vi "CAN2.vi"() -> (0 "error out":errorcluster, 1 "CAN 2":T1, 2 "CAN1":T1, 3 "FPGA VI Reference Out":refnum<k20>)   [LabVIEW 2021]
uses:
  <vilib>/FPGAPlugInAG/cRIO-9068/niLvFpga_Open_cRIO-9068.vi
  <vilib>/FPGAPlugInAG/cRIO-9068/niLvFpga_Run_cRIO-9068.vi
  <vilib>/xnet/xnet.llb/XNET Create Session (Frame Input Stream).vi
  <vilib>/xnet/xnet.llb/XNET Create Session (Frame Output Stream).vi
  <vilib>/rvi/interface/nirviOpenFPGA/nirviOpenFPGA.xnode
  FPGA Bitfiles/pv-emulators_FPGATarget_emptyFPGA_z5uule7UYNw.lvbitx
  <vilib>/rvi/interface/nirviMethod/nirviMethod.xnode
  <resource>/objmgr/xnet.rc
panel:
  out "Devices":refnum<k21>[](array[refnum])
  out "iteration":i32
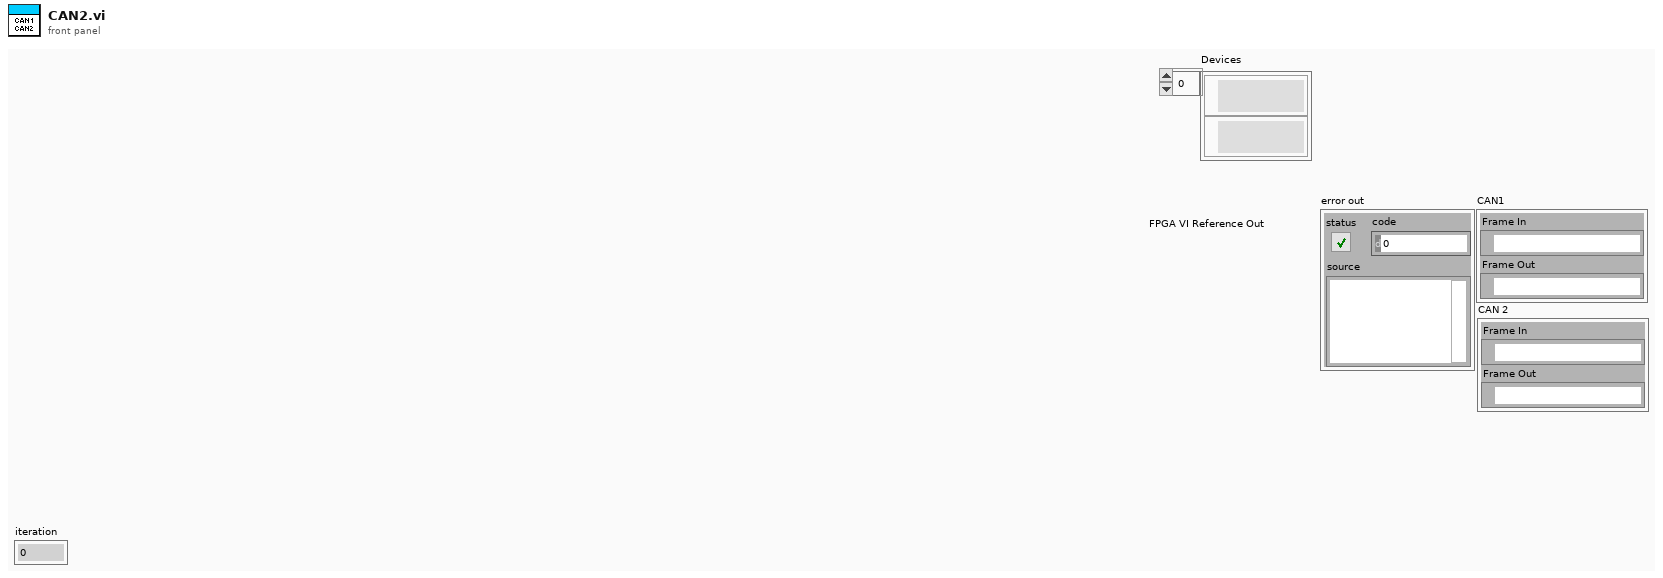
[diagram p1: front panel]
types:
  T1 = cluster{"Frame In":refnum<k21>, "Frame Out":refnum<k21>}
  T2 = cluster{"session out":refnum<k21>, "session out":refnum<k21>}
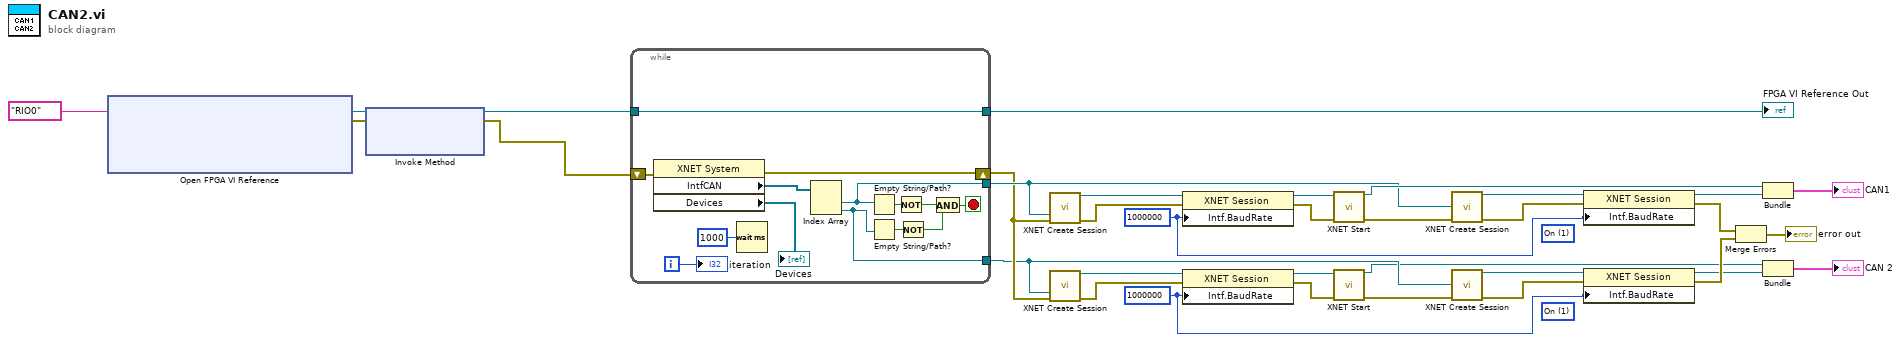
[diagram p0: block diagram]
diagram:
  (unwired) u32 1 items=["Off", "On"] ("Interface:CAN:Termination")
  w4 = u32 1000000 ("y")
  (unwired) u32 1 items=["Off", "On"] ("Interface:CAN:Termination")
  w27 = u32 1000000 ("y")
  n1 = xnode "Open FPGA VI Reference"("resource name"=tag "RIO0") -> ("FPGA VI Reference Out"=w20:refnum<k20>, "error out"=w22:errorcluster)  [unwired: 1 in]
  n2 = xnode "Invoke Method"("FPGA VI Reference In"=w20, "error in"=w22) -> ("FPGA VI Reference Out"=w19:refnum<k20>, "error out"=w18:errorcluster)  [unwired: 1 in]
  n3 = while {
    tunnel: [w41] -> w17
    tunnel: [w45] -> w23
    tunnel: w19 -> [w45]
    shift-right: [w43] -> w16
    shift-left: w18 -> [w44]
    tunnel: [w40] -> w15
    i -> [w47]
    stop <- w35 stop-if-true
    n4 = property class="XNET System"(error in=w44) -> (error out=w43:errorcluster, "IntfCAN"=w42:refnum<k21>[], "Devices"=→"Devices":refnum<k21>[])  [unwired: 1 in, 1 out]
    n5 = Wait (ms)(milliseconds to wait=u32 1000) -> ()  [unwired: 1 out]
    n6 = Index Array(array=w42) -> (element #1=w41:refnum<k21>, element #2=w40:refnum<k21>)  [unwired: 2 in]
    n7 = Empty String/Path?(string/path=w41) -> (empty?=w38:bool)
    n8 = Empty String/Path?(string/path=w40) -> (empty?=w39:bool)
    n9 = Not(x=w38) -> (.not. x?=w37:bool)
    n10 = Not(x=w39) -> (.not. x?=w36:bool)
    n11 = And(x=w37, y=w36) -> (x .and. y?=w35:bool)
    "iteration" <- w47
  }
  "FPGA VI Reference Out" <- w23
  n12 = call-poly <vilib>:"XNET Create Session.vi"("interface"=w17, "error in (no error)"=w16) -> ("session out"=w32:refnum<k21>, "error out"=w33:errorcluster)  [unwired: 12 out]
  n13 = call-poly <vilib>:"XNET Create Session.vi"("interface"=w15, "error in (no error)"=w16) -> ("session out"=w9:refnum<k21>, "error out"=w10:errorcluster)  [unwired: 12 out]
  n14 = property class="XNET Session"(reference=w32, error in=w33, "Intf.BaudRate"=w27) -> (reference out=w31:refnum<k21>, error out=w30:errorcluster)
  n15 = property class="XNET Session"(reference=w9, error in=w10, "Intf.BaudRate"=w4) -> (reference out=w8:refnum<k21>, error out=w7:errorcluster)
  n16 = call <vilib>:"XNET Start.vi"("session in"=w31, "error in (no error)"=w30) -> ("session out"=w25:refnum<k21>, "error out"=w29:errorcluster)  [unwired: 12 out]
  n17 = call <vilib>:"XNET Start.vi"("session in"=w8, "error in (no error)"=w7) -> ("session out"=w3:refnum<k21>, "error out"=w6:errorcluster)  [unwired: 12 out]
  n18 = call-poly <vilib>:"XNET Create Session.vi"("interface"=w17, "error in (no error)"=w29) -> ("session out"=w34:refnum<k21>, "error out"=w28:errorcluster)  [unwired: 1 in, 11 out]
  n19 = call-poly <vilib>:"XNET Create Session.vi"("interface"=w15, "error in (no error)"=w6) -> ("session out"=w11:refnum<k21>, "error out"=w5:errorcluster)  [unwired: 1 in, 11 out]
  n20 = property class="XNET Session"(reference=w34, error in=w28, "Intf.BaudRate"=w27) -> (reference out=w24:refnum<k21>, error out=w14:errorcluster)
  n21 = property class="XNET Session"(reference=w11, error in=w5, "Intf.BaudRate"=w4) -> (reference out=w2:refnum<k21>, error out=w13:errorcluster)
  n22 = Merge Errors(w14, w13) -> (→"error out":errorcluster)
  n23 = Bundle("session out"=w25, "session out"=w24) -> (→"CAN1":T2)  [unwired: 1 in]
  n24 = Bundle("session out"=w3, "session out"=w2) -> (→"CAN 2":T2)  [unwired: 1 in]
